vi "releaseRefArray.vi"(8 "error in (no error)":errorcluster, 11 "IBaseObject in":refnum<class "IBaseObject.lvclass">[](array[class])) -> (0 "error out":errorcluster)   [LabVIEW 2022 SP3, in "openDAQ.lvlib" / "IBaseObject.lvlib" / "IBaseObject.lvclass"]
uses:
  <instrlib>/openDAQ/Public/Classes/IBaseObject/IBaseObject.lvclass
  <instrlib>/openDAQ/Public/Classes/IBaseObject/IBaseObject.lvclass/IBaseObject.ctl
  <instrlib>/openDAQ/Binaries/Windows/x86/copendaq32.dll
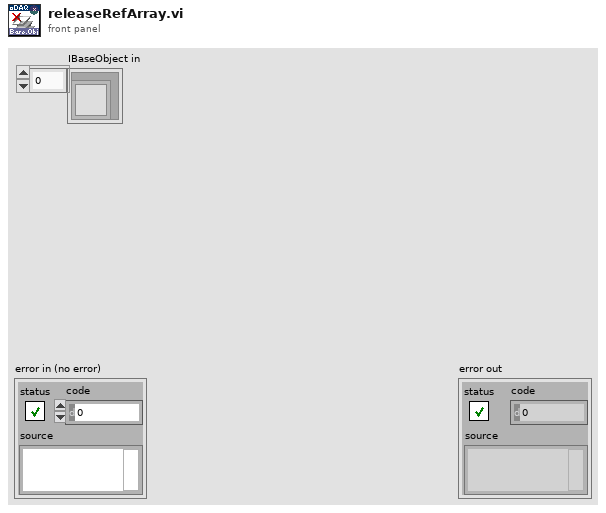
[diagram p1: front panel]
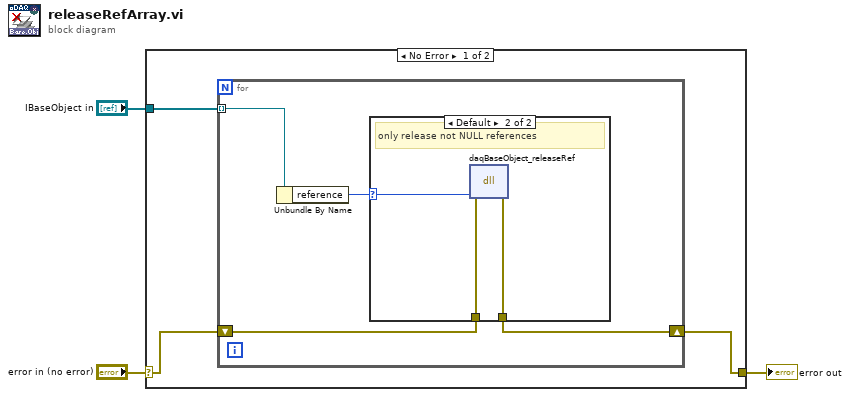
[diagram p0: block diagram]
diagram:
  n1 = case shown="No Error" "error in (no error)" {
    selector: "error in (no error)" -> [w6 w15]
    tunnel: [w5 w15] -> w2
    tunnel: "IBaseObject in" -> [w4 _]
    frame No Error {
      n2 = for {
        shift-right: [w9] -> w5
        shift-left: w6 -> [w10]
        tunnel: w4 -> [w7] mode=indexing
        n3 = Unbundle By Name(w7) -> ("reference"=w8:i64)
        n4 = case shown="Default" w8 {
          selector: w8 -> [_ w12]
          tunnel: w10 -> [w11 w14]
          tunnel: [w11 w13] -> w9
          frame 0 {
          }
          frame Default {
            # "only release not NULL references"
            n5 = dll-call lib="C:/Program Files (x86)/National Instruments/LabVIEW 2022/instr.lib/openDAQ/Binaries/Windows/x86/copendaq*.*" fn="daqBaseObject_releaseRef"(error in=w14, "reference"=w12) -> (error out=w13:errorcluster)  [unwired: 4 in, 1 out]
          }
        }
      }
    }
    frame Error {
    }
  }
  "error out" <- w2
